vi "Volume Accounting.vi"(6 "Reset Volume Counter (T)":bool=TRUE, 7 "Pump ID (0:A)":T1, 8 "error in (no error)":errorcluster, 11 "VISA resource in":refnum<visa-resource-name>) -> (0 "error out":errorcluster, 3 "VISA resource out":refnum<visa-resource-name>)   [LabVIEW 2020, in "Global FIA milliGAT.lvlib"]
doc: "Updates the total amount of volume that has been pumped by the pump."
uses:
  <instrlib>/RxnRover/Global FIA milliGAT 3.14/Global FIA milliGAT.lvlib
  <instrlib>/RxnRover/Global FIA milliGAT 3.14/Public/Utility/Pump Address.ctl
  <instrlib>/RxnRover/Global FIA milliGAT 3.14/Private/Pump Parameter.ctl
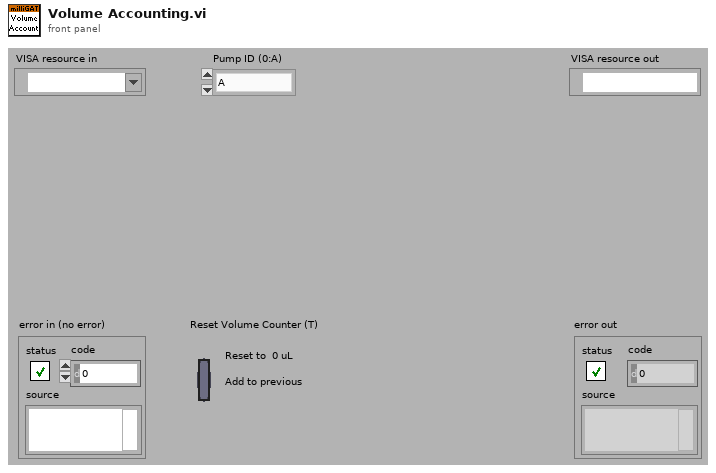
[diagram p1: front panel]
types:
  T1 = typedef "Global FIA milliGAT.lvlib/Pump Address.ctl" = enum16{"A", "B", "C", "D", "E", "F", "G", "H", "I", "J", "K", "L", "M", "N", "O", "P", "Q", "R", "S", "T", "U", "V", "W", "X", "Y", "Z", "a", "b", "c", "d", "e", "f", "g", "h", "i", "j", "k", "l", "m", "n", "o", "p", "q", "r", "s", "t", "u", "v", "w", "x", "y", "z", "0", "1", "2", "3", "4", "5", "6", "7", "8", "9"}
  T2 = typedef "Global FIA milliGAT.lvlib/Pump Parameter.ctl" = enum16{"Enabled", "EU", "EU Calibration Factor", "Fixed Asp or Disp", "Starting Position", "Starting Flow", "Peak Flow", "Flow Acceleration", "Flow Deceleration", "Session Volume", "Max Pressure", "Backlash (usteps)", "BL Calibration Factor", "BL Correction Enabled", "Min Flow", "Max Flow", "Min Acceleration", "Max Acceleration", "Service Volume", "Life Volume"}
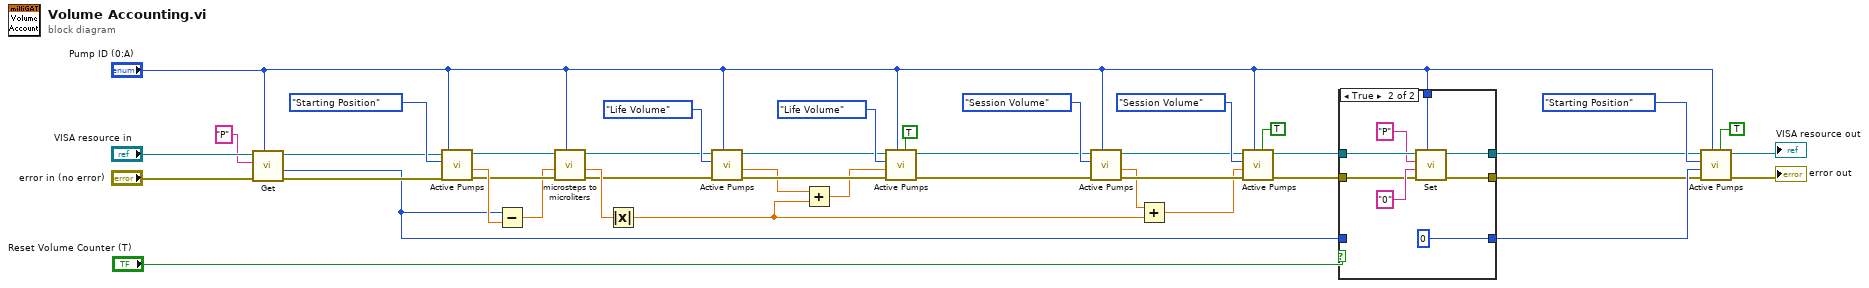
[diagram p0: block diagram]
diagram:
  n1 = call <instrlib>:"Get.vi"("Pump ID (0:A)"="Pump ID (0:A)", "error in (no error)"="error in (no error)", "Parameter"="P" ("Parameter or Flag"), "VISA resource in"="VISA resource in") -> ("error out"=w22:errorcluster, "Value"=w14:i32, "VISA resource out"=w23:refnum<visa-resource-name>)  [unwired: 5 in]
  n2 = call <instrlib>:"Active Pumps.vi"("Pump ID (0:A)"="Pump ID (0:A)", "error in (no error)"=w22, "Parameter"=Pump_Parameter."Starting Position", "VISA resource in"=w23) -> ("error out"=w27:errorcluster, "Value out"=w28:dbl, "VISA resource out"=w26:refnum<visa-resource-name>)  [unwired: 4 in, 1 out]
  n3 = Subtract(x=w14, y=w28) -> (x-y=w15:dbl)
  n4 = call <instrlib>:"microsteps to microliters.vi"("Pump ID (0:A)"="Pump ID (0:A)", "error in (no error)"=w27, "Microsteps (0)"=w15, "VISA resource in"=w26) -> ("error out"=w12:errorcluster, "Microliters"=w17:dbl, "VISA resource out"=w11:refnum<visa-resource-name>)  [unwired: 5 in]
  n5 = Absolute Value(x=w17) -> (abs(x)=w2:dbl)
  n6 = call <instrlib>:"Active Pumps.vi"("Pump ID (0:A)"="Pump ID (0:A)", "error in (no error)"=w12, "Parameter"=Pump_Parameter."Life Volume", "VISA resource in"=w11) -> ("error out"=w7:errorcluster, "Value out"=w3:dbl, "VISA resource out"=w8:refnum<visa-resource-name>)  [unwired: 4 in, 1 out]
  n7 = Add(x=w3, y=w2) -> (x+y=w1:dbl)
  n8 = call <instrlib>:"Active Pumps.vi"("Action (F:Read)"=TRUE, "Pump ID (0:A)"="Pump ID (0:A)", "error in (no error)"=w7, "Value in"=w1, "Parameter"=Pump_Parameter."Life Volume", "VISA resource in"=w8) -> ("error out"=w4:errorcluster, "VISA resource out"=w5:refnum<visa-resource-name>)  [unwired: 2 in, 2 out]
  n9 = call <instrlib>:"Active Pumps.vi"("Pump ID (0:A)"="Pump ID (0:A)", "error in (no error)"=w4, "Parameter"=Pump_Parameter."Session Volume", "VISA resource in"=w5) -> ("error out"=w36:errorcluster, "Value out"=w33:dbl, "VISA resource out"=w35:refnum<visa-resource-name>)  [unwired: 4 in, 1 out]
  n10 = Add(x=w33, y=w2) -> (x+y=w16:dbl)
  n11 = call <instrlib>:"Active Pumps.vi"("Action (F:Read)"=TRUE, "Pump ID (0:A)"="Pump ID (0:A)", "error in (no error)"=w36, "Value in"=w16, "Parameter"=Pump_Parameter."Session Volume", "VISA resource in"=w35) -> ("error out"=w19:errorcluster, "VISA resource out"=w21:refnum<visa-resource-name>)  [unwired: 2 in, 2 out]
  n12 = case shown="True" "Reset Volume Counter (T)" {
    tunnel: w19 -> [w44 w49]
    tunnel: w21 -> [w45 w53]
    tunnel: "Pump ID (0:A)" -> [_ w52]
    tunnel: [w45 w48] -> w20
    tunnel: [w44 w47] -> w18
    tunnel: [w43 0 ("Value")] -> w31
    tunnel: w14 -> [w43 _]
    frame False {
    }
    frame True {
      n13 = call <instrlib>:"Set.vi"("Pump ID (0:A)"=w52, "error in (no error)"=w49, "Expression"="0", "Parameter"="P", "VISA resource in"=w53) -> ("error out"=w47:errorcluster, "VISA resource out"=w48:refnum<visa-resource-name>)  [unwired: 5 in]
    }
  }
  n14 = call <instrlib>:"Active Pumps.vi"("Action (F:Read)"=TRUE, "Pump ID (0:A)"="Pump ID (0:A)", "error in (no error)"=w18, "Value in"=w31, "Parameter"=Pump_Parameter."Starting Position", "VISA resource in"=w20) -> ("error out"=→"error out":errorcluster, "VISA resource out"=→"VISA resource out":refnum<visa-resource-name>)  [unwired: 2 in, 2 out]
